vi "DS345.set phase.vi"(0 "i ref in":refnum<vi>, 2 "phase [degree]":dbl min=0.0 max=1500.0 step=1.0 format="%.3f", 5 "error in (no error)":errorcluster) -> (14 "i ref out":refnum<vi>, 19 "error out":errorcluster)   [LabVIEW 2014, in "DS345.lvlib"]
doc: "sets the phase for a DS345."
uses:
  DS345.lvlib
  CSCore/CSSystem/CoreLib/CoreLib.lvlib
  CSCore/CSSystem/CoreDefs/CoreDefs.error_type.ctl
  CSCore/CSApplicationBaseClasses/DeviceBase/DeviceBase.lvlib
  CSCore/CSApplicationBaseClasses/AFGBase/AFGBase.lvlib
  CSCore/CSApplicationBaseClasses/AFGBase/AFGBase.directionType.ctl
  CSCore/CSApplicationBaseClasses/AFGBase/AFGBase.serviceType.ctl
  CSlibraries/UtilityLib/UtilityLib.valueStatus.ctl
  CSlibraries/UtilityLib/UtilityLib.lvlib
  CSCore/CSApplicationBaseClasses/DeviceBase/DeviceBase.deviceState.ctl
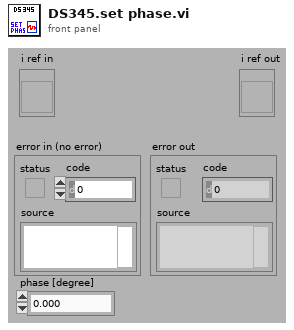
[diagram p1: front panel]
types:
  T1 = typedef "AFGBase.lvlib/AFGBase.serviceType.ctl" = enum16{"frequency", "amplitude", "phase", "DCOffset", "enableOutput", "trigger", "waveformType"}
  T2 = typedef "AFGBase.lvlib/AFGBase.directionType.ctl" = enum16{"unknown", "update actual value", "update nominal value", "update both"}
  T3 = typedef "UtilityLib.lvlib/UtilityLib.valueStatus.ctl" = enum16{"no info available", "stand by/off", "on", "warning", "alarm/malfunction", "not implemented", "user action required", "important information", "system default", "control default", "indicator default", "button default"}
  T4 = typedef "CoreDefs.error_type.ctl" = enum16{"no error", "can't load process", "can't unload process", "process does not exist", "can't install process", "can't remove process", "unknown function", "time out", "can't execute function", "duplicate queue name", "super not found", "caller queue invalid", "can't ping process", "unknown error", "VISA Error", "VISA timeout", "GPIB timeout", "GPIB error", "communication error", "data type mismatch", "can't read data from OPC server", "can't write data to OPC server", "OET error", "function not implemented", "process already exists", "invalid Shared Variable name", "error writing Shared Variable", "error reading Shared Variable", "invalid client name", "corrupt database", "unknown class", "call not authorized", "parameter out of range", "OET timeout: can't get data to modify", "invalid queue name", "requested operation incompatible with current state", "event undefined", "event disabled", "state undefined", "caller is not a friend", "EventBuilder: bad eventID", "EventBuilder: no DAQ devices", "a thread must not stop itself", "UNUSED ELEMENT4", "DiscArchiver: eventData incomplete", "DiscArchiver: eventData does not belong to run", "DiscArchiver: can't open file", "DiscArchiver: can't write to file", "DiscArchiver: available disc space low", "can't acquire semaphore", "error reading data from database", "notifier object is not existing", "can't register process", "can't unregister process", "illegal event type", "object disabled", "object already exists", "can't change state", "Instrument not found", "no connection to remote node", "invalid reference", "N/A", "UNUSED ELEMENT 1", "element not found", "illegal TCP/IP connection detected", "object does not exist", "invalid access ID", "unknown CS system", "invalid privilige", "unsupported data type", "unsupported server type", "IO server already exists", "Shared Variable already exists"}
  T5 = typedef "DeviceBase.lvlib/DeviceBase.deviceState.ctl" = i16
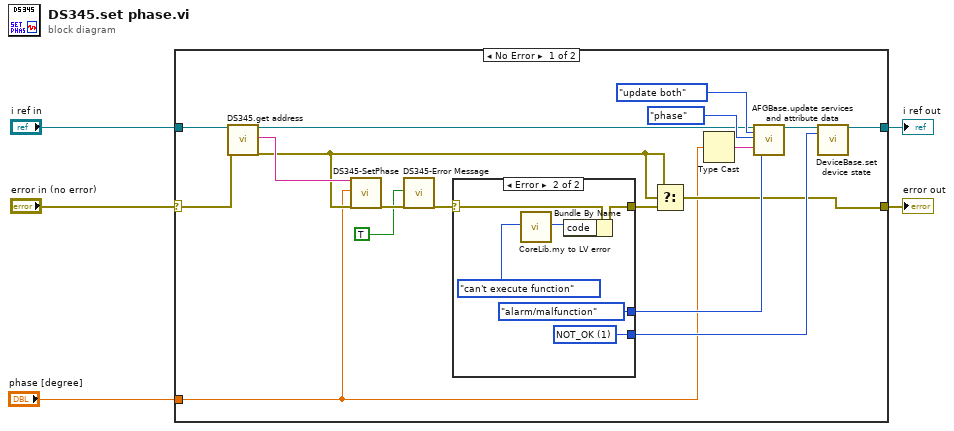
[diagram p0: block diagram]
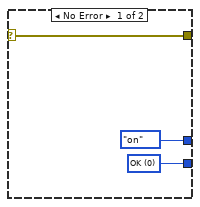
[diagram p2: hidden frame]
diagram:
  n1 = case shown="No Error" "error in (no error)" {
    selector: "error in (no error)" -> [w16 w33]
    tunnel: [w8 w33] -> w5
    tunnel: "phase [degree]" -> [w6 _]
    tunnel: "i ref in" -> [w22 w34]
    tunnel: [w11 w34] -> w2
    frame No Error {
      n2 = call "DS345.get address.vi"("i ref in"=w22, "error in (no error)"=w16) -> ("i ref out"=w12:refnum<vi>, "address"=w23:string, "error out"=w21:errorcluster)  [unwired: 15 in]
      n3 = call "DS345-SetPhase.vi"("address string"=w23, "phase"=w6, "error in (no error)"=w21) -> ("error out"=w20:errorcluster)  [unwired: 15 in, 1 out]
      n4 = call "DS345-Error Message.vi"("addMessageToSource"=TRUE ("add message to source"), "error in (no error)"=w20) -> ("error out"=w19:errorcluster)  [unwired: 14 in, 3 out]
      n5 = case shown="Error" w19 {
        selector: w19 -> [w26 w32]
        tunnel: [w26 w31] -> w17
        tunnel: [UtilityLib.valueStatus."on" ("quality") UtilityLib.valueStatus."alarm/malfunction" ("quality")] -> w10
        tunnel: [w24 w27] -> w9
        frame No Error {
          w24 = T5 0 items=["ERROR"=-1, "OK"=0, "NOT_OK"=1] ("deviceState")
        }
        frame Error {
          w27 = T5 1 items=["ERROR"=-1, "OK"=0, "NOT_OK"=1] ("deviceState")
          n6 = call "CoreLib.my to LV error.vi"("ErrorTypes"=CoreDefs.error_type."can't execute function") -> ("LV error code"=w30:i32)  [unwired: 17 in, 1 out]
          n7 = Bundle By Name(cluster=w32, "code"=w30) -> (w31:errorcluster)
        }
      }
      n8 = Select(t=w21, s=w21, f=w17) -> (s? t:f=w8:errorcluster)
      n9 = Type Cast(x=w6) -> (*(type *) &x=w7:string)  [unwired: 1 in]
      n10 = call "AFGBase.update services and attribute data.vi"("i ref in"=w12, "direction"=AFGBase.directionType."update both", "service"=AFGBase.serviceType."phase", "value"=w7, "quality"=w10) -> ("i ref out"=w15:refnum<vi>)  [unwired: 12 in, 2 out]
      n11 = call "DeviceBase.set device state.vi"("i ref in"=w15, "deviceState"=w9) -> ("i ref out"=w11:refnum<vi>)  [unwired: 15 in, 2 out]
    }
    frame Error {
    }
  }
  "error out" <- w5
  "i ref out" <- w2
